vi "Read.vi"(7 "I2C Channel (0)":u8, 8 "Error In":errorcluster, 11 "LINX Resource":T1) -> (0 "Error Out":errorcluster, 2 "Compass (Gauss)":cluster{"X":dbl, "Y":dbl, "Z":dbl}, 3 "LINX Resource":T1)   [LabVIEW 2014, in "LMH-LINX.lvlib" / "PmodCMPS.lvlib"]
doc: "Read X, Y and Z axis data from the PmodCMPS and return values as Gauss."
uses:
  PmodCMPS.lvlib
  Private/Type Defs/LINX Ref.ctl
  Private/Type Defs/Platform.ctl
  Private/Type Defs/Interface.ctl
  Private/Device/Type Defs/LINX Device Config.ctl
  Private/Device/Type Defs/TCP Config.ctl
  Private/Device/Type Defs/Channels.ctl
  LMH-LINX.lvlib
  <vilib>/MakerHub/Toolbox/LMH-Toolbox.lvlib
  Private/Device/Device.lvlib
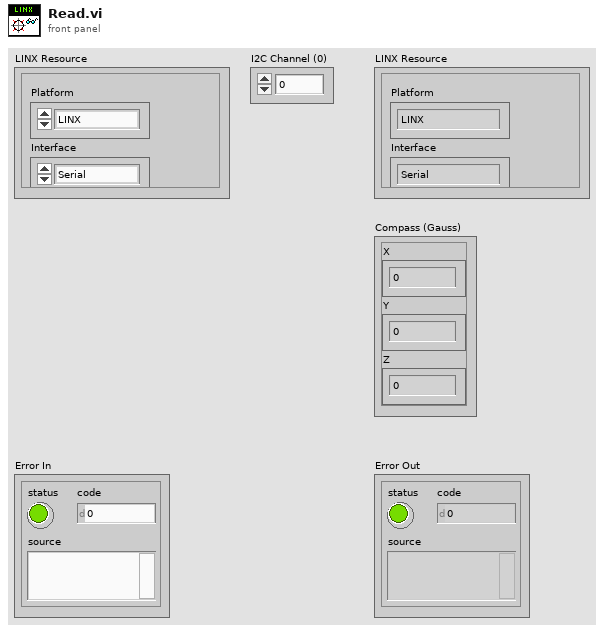
[diagram p1: front panel]
types:
  T1 = typedef "LMH-LINX.lvlib/LINX Ref.ctl" = cluster{"Platform":T2, "Interface":T3, "LINX Device Config":T4}
  T2 = typedef "LMH-LINX.lvlib/Platform.ctl" = enum16{"LINX", "myRIO"}
  T3 = typedef "LMH-LINX.lvlib/Interface.ctl" = enum16{"Serial", "TCP"}
  T4 = typedef "LMH-LINX.lvlib/Device.lvlib/LINX Device Config.ctl" = cluster{"Interface":T3, "COM Port":refnum<visa-resource-name>, "TCP Configuration":T5, "Device Family":u8, "Device ID":u8, "Device Name":string, "TCP Ref":refnum<k5>, "Channels":T6}
  T5 = typedef "LMH-LINX.lvlib/Device.lvlib/TCP Config.ctl" = cluster{"IP Address":string, "Port":u16}
  T6 = typedef "LMH-LINX.lvlib/Channels.ctl" = cluster{"DI":u8[], "DO":u8[], "AI":u8[], "AO":u8[], "PWM":u8[], "QE":u8[], "UART":u8[], "I2C 2":u8[], "SPI":u8[], "CAN":u8[], "Servo":u8[], "AI Ref (V)":dbl, "AO Ref (V)":dbl, "AO Resolution (Bits)":u8}
  T7 = cluster{"Decimal I16":i16, "Decimal I16":i16, "Decimal I16":i16}
  T8 = cluster{"Decimal I16":dbl, "Decimal I16":dbl, "Decimal I16":dbl}
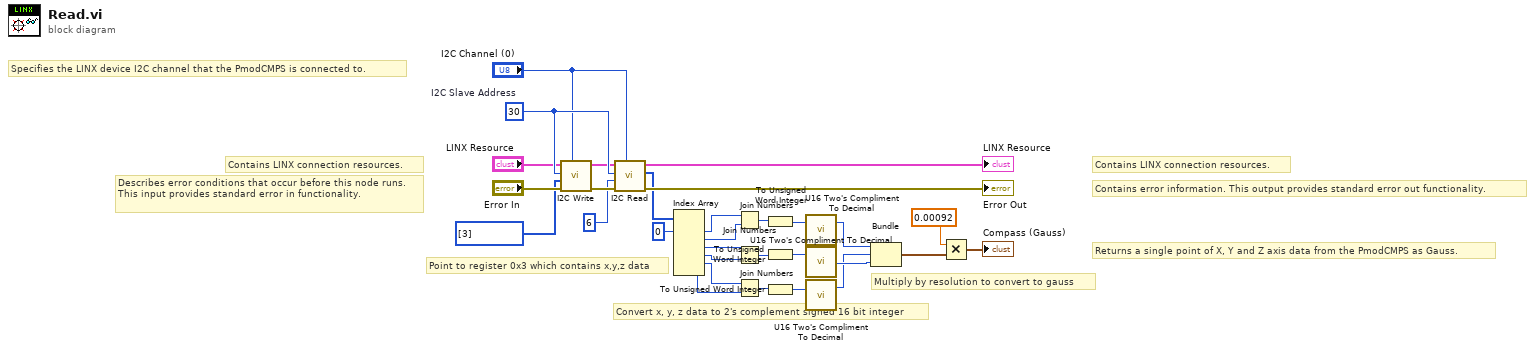
[diagram p0: block diagram]
diagram:
  w30 = u8 30  # I2C Slave Address
  # "Returns a single point of X, Y and Z axis data from the PmodCMPS as Gauss."
  # "Specifies the LINX device I2C channel that the PmodCMPS is connected to."
  # "Contains LINX connection resources."
  # "Contains error information. This output provides standard error out functionality."
  # "Contains LINX connection resources."
  # "Describes error conditions that occur before this node runs. This input provides standard error in functionality."
  # "Multiply by resolution to convert to gauss"
  # "Convert x, y, z data to 2's complement signed 16 bit integer"
  # "Point to register 0x3 which contains x,y,z data"
  n1 = call "I2C Write.vi"("I2C Channel"="I2C Channel (0)", "Error In"="Error In", "Data"=u8[] [3], "I2C Slave Address (0)"=w30, "LINX Resource"="LINX Resource") -> ("Error Out"=w6:errorcluster, "LINX Resource"=w5:T1)  [unwired: 5 in]
  n2 = call "I2C Read.vi"("I2C Channel"="I2C Channel (0)", "Error In"=w6, "Bytes To Read"=u8 6, "I2C Slave Address (0)"=w30, "LINX Resource"=w5) -> ("Error Out"=→"Error Out":errorcluster, "Data"=w9:u8[], "LINX Resource"=→"LINX Resource":T1)  [unwired: 4 in]
  n3 = Index Array(array=w9, index #1=0 ("index")) -> (element #1=w24:u8, element #2=w25:u8, element #3=w26:u8, element #4=w27:u8, element #5=w28:u8, element #6=w29:u8)  [unwired: 5 in]
  n4 = Join Numbers(hi=w24, lo=w25) -> ((hi.lo)=w11:u16)
  n5 = Join Numbers(hi=w26, lo=w27) -> ((hi.lo)=w12:u16)
  n6 = Join Numbers(hi=w28, lo=w29) -> ((hi.lo)=w13:u16)
  n7 = To Unsigned Word Integer(number=w11) -> (unsigned 16bit integer=w16:u16)
  n8 = To Unsigned Word Integer(number=w12) -> (unsigned 16bit integer=w14:u16)
  n9 = To Unsigned Word Integer(number=w13) -> (unsigned 16bit integer=w15:u16)
  n10 = call <vilib>:"U16 Two's Compliment To Decimal.vi"("Two's Compliment U16"=w16) -> ("Decimal I16"=w17:i16)  [unwired: 2 in]
  n11 = call <vilib>:"U16 Two's Compliment To Decimal.vi"("Two's Compliment U16"=w14) -> ("Decimal I16"=w23:i16)  [unwired: 2 in]
  n12 = call <vilib>:"U16 Two's Compliment To Decimal.vi"("Two's Compliment U16"=w15) -> ("Decimal I16"=w22:i16)  [unwired: 2 in]
  n13 = Bundle("Decimal I16"=w17, "Decimal I16"=w22, "Decimal I16"=w23) -> (w18:T7)  [unwired: 1 in]
  n14 = Multiply(x=0.00092, y=w18) -> (x*y=→"Compass (Gauss)":T8)
